vi "Check Hierarchy.vi"(8 "error in (no error)":errorcluster, 11 "ExecAnchor in":refnum<class "ExecAnchor.lvclass">) -> (0 "error out":errorcluster, 3 "ExecAnchor out":refnum<class "ExecAnchor.lvclass">)   [LabVIEW 2020, in "ExecAnchor.lvclass"]
uses:
  ExecAnchor.lvclass
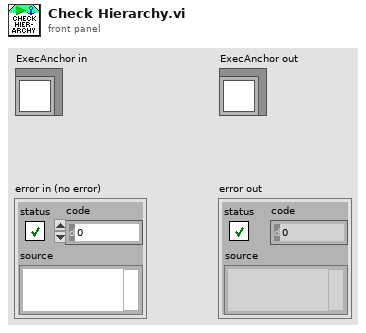
[diagram p1: front panel]
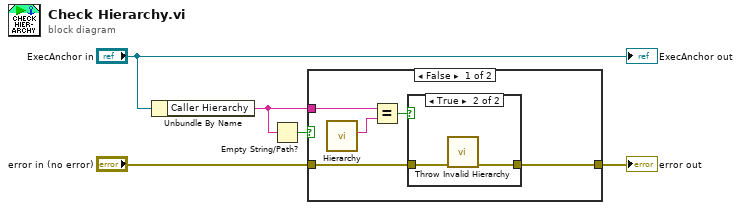
[diagram p0: block diagram]
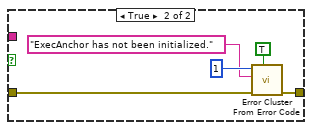
[diagram p3: hidden frame]
diagram:
  n1 = Unbundle By Name("ExecAnchor in") -> ("Caller Hierarchy"=w2:string)
  n2 = Empty String/Path?(string/path=w2) -> (empty?=w3:bool)
  n3 = case shown="False" w3 {
    tunnel: "error in (no error)" -> [w7 w18]
    tunnel: w2 -> [w10 _]
    tunnel: [w6 w17] -> w1
    frame False {
      n4 = call "Hierarchy.vi"() -> ("Hierarchy"=w9:string)  [unwired: 11 in]
      n5 = Equal?(x=w10, y=w9) -> (x = y?=w8:bool)
      n6 = case shown="True" w8 {
        tunnel: w7 -> [w11 w13]
        tunnel: [w11 w12] -> w6
        frame False {
        }
        frame True {
          n7 = call "Throw Invalid Hierarchy.vi"("error in (no error)"=w13) -> ("error out"=w12:errorcluster)  [unwired: 10 in]
        }
      }
    }
    frame True {
      n8 = call <vilib>:"Error Cluster From Error Code.vi"("show call chain? (False)"=TRUE, "error in (no error)"=w18, "error message (\"\")"="ExecAnchor has not been initialized." ("error message (\"\")"), "error code (0)"=1) -> ("error out"=w17:errorcluster)  [unwired: 5 in]
    }
  }
  "error out" <- w1
  "ExecAnchor out" <- "ExecAnchor in"
